vi "TDMSSetSelection.vi"(7 "task":T1(ring), 8 "error in (no error)":errorcluster, 10 "min/max [t, F, z]":dbl[](array[numeric]), 11 "tracename in":string="D:\\current VIs\\Vi\\Data\\data_074.tdms: 20") -> (0 "error out":errorcluster, 2 "Selected":dbl[](graph), 3 "tracename out":string="E:\\current VIs\\Vi\\Data\\data_074.tdms: 20")   [LabVIEW 2018]
panel:
  out "size(s)":i32
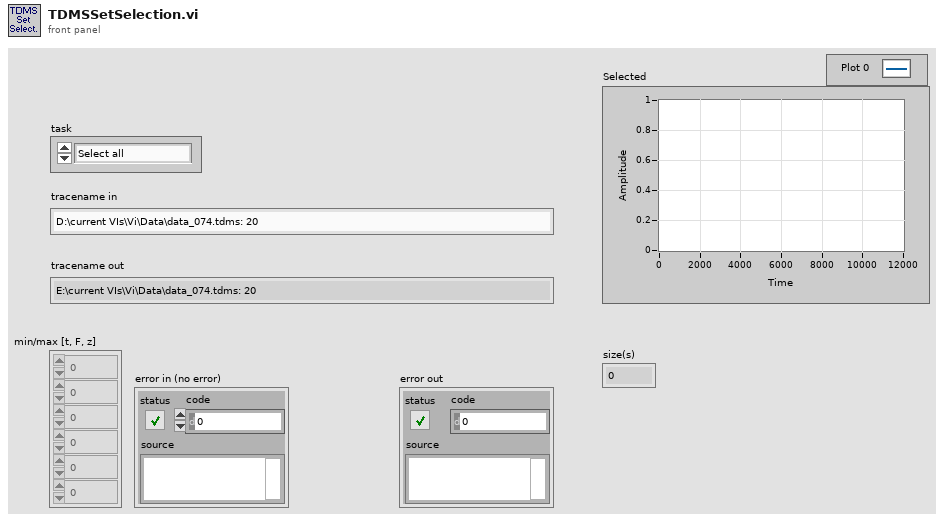
[diagram p1: front panel]
types:
  T1 = enum16{"Select all", "Select none", "Include", "Exclude"}
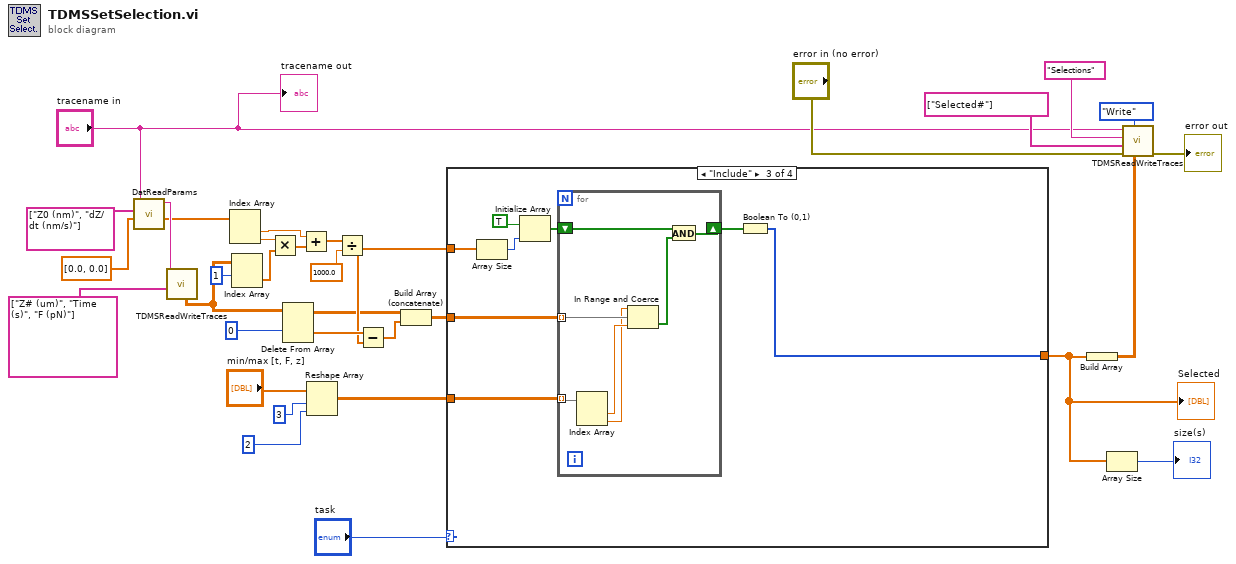
[diagram p0: block diagram]
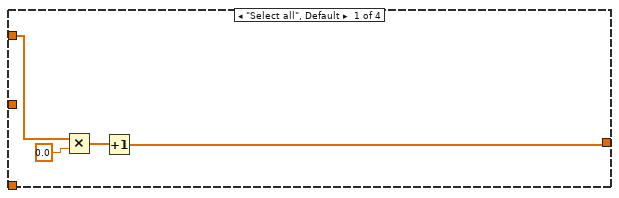
[diagram p2: hidden frame]
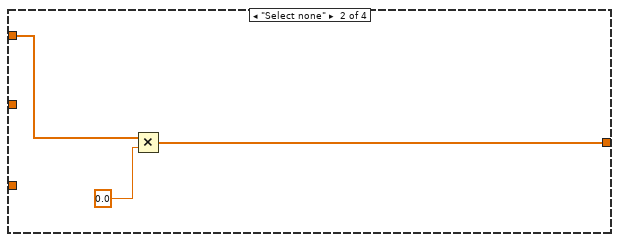
[diagram p3: hidden frame]
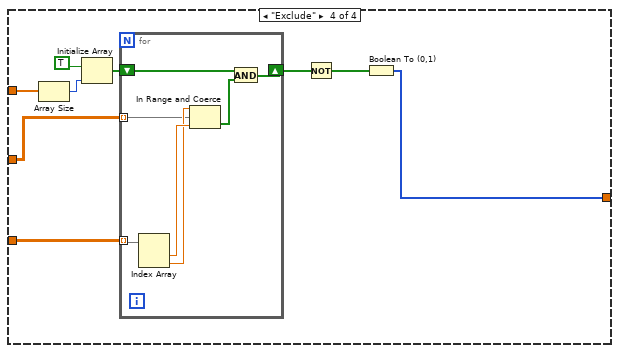
[diagram p4: hidden frame]
diagram:
  n1 = call "DatReadParams.vi"("default Values"=dbl[] [0.0, 0.0] ("Default values"), "Names"=string[] ["Z0 (nm)", "dZ/dt (nm/s)"] ("Par names"), "tracename"="tracename in") -> ("Values out"=w10:dbl[], "tracename out"=w17:string)  [unwired: 4 in, 1 out]
  n2 = call "TDMSReadWriteTraces.vi"("Channels in"=string[] ["Z# (um)", "Time (s)", "F (pN)"] ("channel name(s) in"), "tracename"=w17) -> ("Data out"=w3:dbl[][])  [unwired: 4 in, 5 out]
  n3 = Index Array(array=w10) -> (element #1=w13:dbl, element #2=w15:dbl)  [unwired: 2 in]
  n4 = Index Array(array=w3, index (row)=1) -> (element=w5:dbl[])  [unwired: 1 in]
  n5 = Multiply(x=w15, y=w5) -> (x*y=w14:dbl[])
  n6 = Delete From Array(array=w3, index (row)=0) -> (deleted portion=w8:dbl[], array with subset deleted=w1:dbl[][])  [unwired: 2 in]
  n7 = Add(x=w13, y=w14) -> (x+y=w12:dbl[])
  n8 = Reshape Array("min/max [t, F, z]", 3 ("dimension size"), 2 ("dimension size")) -> (w29:dbl[][])
  n9 = Divide(x=w12, y=1000.0 ("element")) -> (x/y=w7:dbl[])
  n10 = Subtract(x=w8, y=w7) -> (x-y=w6:dbl[])
  n11 = Build Array (concatenate)(w1, w6) -> (w2:dbl[][])
  n12 = case shown="\"Include\"" "task" {
    tunnel: [w34 w38 w41 w59] -> w22
    tunnel: w29 -> [_ _ w48 w64]
    tunnel: w2 -> [_ _ w43 w56]
    tunnel: w7 -> [w35 w39 w42 w57]
    frame "Select all", Default {
      n13 = Multiply(x=w35, y=0.0) -> (x*y=w36:dbl[])
      n14 = Increment(x=w36) -> (x+1=w34:dbl[])
    }
    frame "Select none" {
      n15 = Multiply(x=w39, y=0.0) -> (x*y=w38:dbl[])
    }
    frame "Include" {
      n16 = Array Size(array=w42) -> (size(s)=w47:i32)
      n17 = Initialize Array(TRUE, w47) -> (w46:bool[])
      n18 = for {
        tunnel: w43 -> [w55] mode=indexing
        tunnel: w48 -> [w54] mode=indexing
        shift-right: [w50] -> w44
        shift-left: w46 -> [w51]
        n19 = Index Array(array=w54) -> (element #1=w53:dbl, element #2=w52:dbl)  [unwired: 2 in]
        n20 = In Range and Coerce(upper limit=w52, x=w55, lower limit=w53) -> (In Range?=w49:bool[])  [unwired: 1 out]
        n21 = And(x=w51, y=w49) -> (x .and. y?=w50:bool[])
      }
      n22 = Boolean To (0,1)(Boolean=w44) -> (0, 1=w41:i16[])
    }
    frame "Exclude" {
      n23 = Array Size(array=w57) -> (size(s)=w63:i32)
      n24 = Initialize Array(TRUE, w63) -> (w62:bool[])
      n25 = for {
        tunnel: w56 -> [w65] mode=indexing
        tunnel: w64 -> [w71] mode=indexing
        shift-right: [w66] -> w60
        shift-left: w62 -> [w67]
        n26 = Index Array(array=w71) -> (element #1=w70:dbl, element #2=w69:dbl)  [unwired: 2 in]
        n27 = In Range and Coerce(upper limit=w69, x=w65, lower limit=w70) -> (In Range?=w68:bool[])  [unwired: 1 out]
        n28 = And(x=w67, y=w68) -> (x .and. y?=w66:bool[])
      }
      n29 = Not(x=w60) -> (.not. x?=w58:bool[])
      n30 = Boolean To (0,1)(Boolean=w58) -> (0, 1=w59:i16[])
    }
  }
  "Selected" <- w22
  n31 = Build Array(w22) -> (w24:dbl[][])
  n32 = Array Size(array=w22) -> (size(s)=→"size(s)":i32)
  n33 = call "TDMSReadWriteTraces.vi"("Data in"=w24, "Task"=enum16{"Read", "Write"}."Write", "error in (no error)"="error in (no error)", "Channels in"=string[] ["Selected#"], "group name"="Selections", "tracename"="tracename in") -> ("error out"=→"error out":errorcluster)  [unwired: 5 out]
  "tracename out" <- "tracename in"
